vi "Get License Type.vi"(8 "error in (no error)":errorcluster, 11 "Engine in":refnum<class "Engine.lvclass">) -> (0 "error out":errorcluster, 2 "TS License Type":T1, 3 "Engine out":refnum<class "Engine.lvclass">)   [LabVIEW 2020, in "TSnax.lvlib" / "Engine.lvclass"]
uses:
  Engine.lvclass
  TS License Type.ctl
  Engine.lvclass/Engine.ctl
  TSnax.lvlib
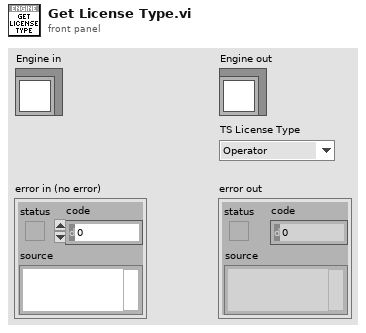
[diagram p1: front panel]
types:
  T1 = typedef "TSnax.lvlib/TS License Type.ctl" = enum16{"Operator", "CustomEditor", "SequenceEditor"}
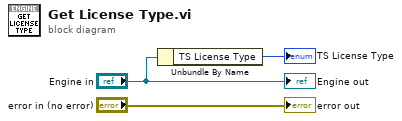
[diagram p0: block diagram]
diagram:
  n1 = Unbundle By Name("Engine in") -> ("TS License Type"=→"TS License Type":T1)
  "error out" <- "error in (no error)"
  "Engine out" <- "Engine in"
